vi "Reset.vi"(8 "error in (no error)":errorcluster, 11 "Contador in":refnum<class "Contador.lvclass">) -> (0 "error out":errorcluster, 3 "Contador out":refnum<class "Contador.lvclass">)   [LabVIEW 2020, in "Contador.lvlib" / "Contador.lvclass"]
uses:
  Contador.lvclass
  Contador.lvclass/Contador.ctl
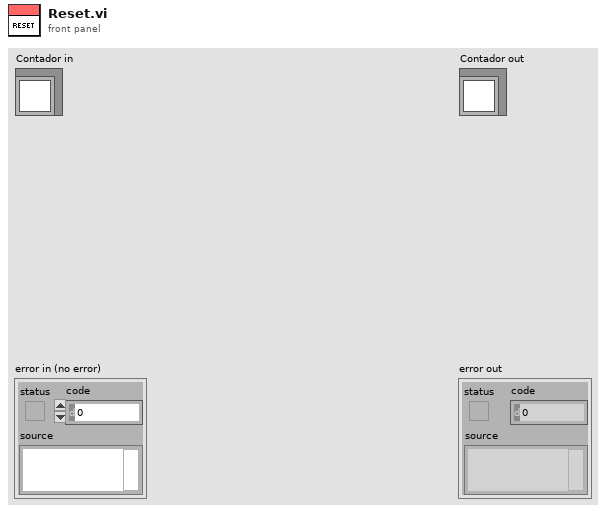
[diagram p1: front panel]
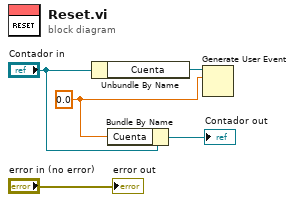
[diagram p0: block diagram]
diagram:
  w1 = 0.0 ("Cuenta")
  n1 = Unbundle By Name("Contador in") -> ("Cuenta"=w3:refnum<user-event>)
  n2 = Bundle By Name(cluster="Contador in", "Cuenta"=w1) -> (→"Contador out":refnum<class "Contador.lvclass">)
  n3 = Generate User Event(user event=w3, event data cluster=w1) -> ()  [unwired: 2 in, 2 out]
  "error out" <- "error in (no error)"
